vi "SMO.UI_Embed.ReftoDVR.vi"(10 "Ref":u32 format="%08x") -> (2 "Ref":T1)   [LabVIEW 2019, in "SMO.UI_Embed.lvclass"]
uses:
  SMO.UI_Embed.lvclass
  Typedefs/PrivateData--Ref.ctl
  Typedefs/PrivateData--Cluster.ctl
  Typedefs/PublicEvents--Cluster.ctl
  Typedefs/SMO.UI_Embed State--enum.ctl
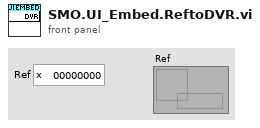
[diagram p1: front panel]
types:
  T1 = typedef "SMO.UI_Embed.lvclass/PrivateData--Ref.ctl" = refnum<data-value>
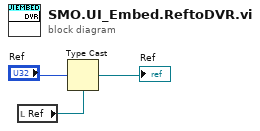
[diagram p0: block diagram]
diagram:
  n1 = local read "Ref"() -> (w1:T1)
  n2 = Type Cast(type=w1, x="Ref") -> (*(type *) &x=→"Ref":T1)
